vi "Laser Feedback-noglobalpower.vi"() -> ()   [LabVIEW 2014]
doc: "This VI first scan 0.1-5 V AOM voltage range 3 times, and use these data to generate a calibration curve. The calibration curve is fitted as a 3 th order polynomial curve, and then passed to the second part. \nSecond, the feedback loop is turned on and PID controller is used to stabilize the intensity.\n\nThis VI includes the following subVI:\n1. (SubVI)AOMvolt-Power Calibration.vi\n2. AOM PID feedback-simplePID(SubVI).vi"
uses:
  <vilib>/Analysis/polynomials.llb/Scalar Polynomial Evaluation (DBL).vi
  <vilib>/addons/control/pid/pid.llb/PID (DBL).vi
  <vilib>/Utility/file.llb/Write To Spreadsheet File (DBL).vi
  <vilib>/Analysis/NI_AALPro.lvlib
  <vilib>/addons/control/pid/NI_PID_pid.lvlib
panel:
  in  "Tab Control":enum32{"Calibration curve", "Power readout"}(tab)
  out "PW-AOM Graph":T1(graph)
  out "Waveform Chart":dbl(graph)
  out "Polynomial Coefficients":dbl[](array[numeric])
  out "AOM (V)":dbl format="%.2f"
  in  "Set Laser power":dbl
  out "Powermeter readout (mW)":dbl
  in  "Save Button":bool
  in  "PID gains 2":T2={"proportional gain (Kc)"=0.0091, "integral time (Ti, min)"=5e-06, "derivative time (Td, min)"=0.0014} {"derivative time (Td, min)" format="%#.6g"; "integral time (Ti, min)" format="%#.6g"; "proportional gain (Kc)" format="%#.6g"}
  in  "stop":bool
  in  "millisecond multiple":u32=5
  out "Start Calibrate":bool
  # "Kc=0.0151\nTi=2.1E-6\nTd=0.0093\n\nKc=0.0151\nTi=5E-6\nTd=0.0014"
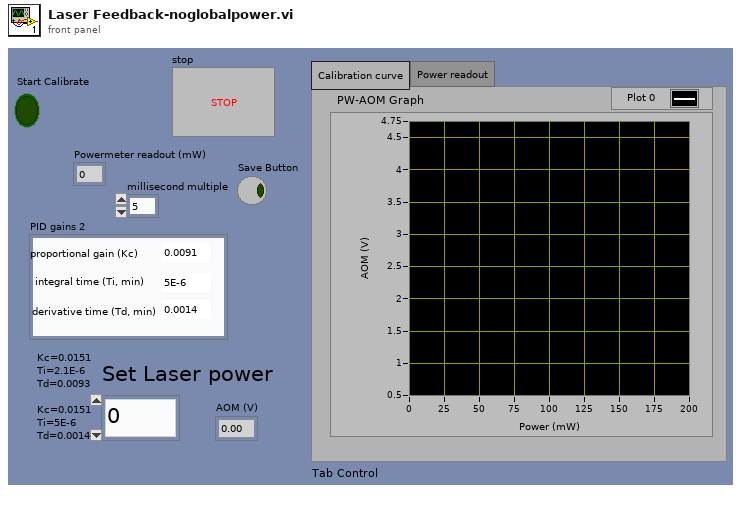
[diagram p1: front panel]
types:
  T1 = cluster{"Cal-PD (mV)":dbl[], "Cal-AOM (V)":dbl[]}[]
  T2 = cluster{"proportional gain (Kc)":dbl, "integral time (Ti, min)":dbl, "derivative time (Td, min)":dbl}
  T3 = cluster{"Cal-PD (mV)":dbl[], "Cal-AOM (V)":dbl[], "Best Polynomial Fit":dbl[], "Polynomial Coefficients":dbl[]}
  T4 = cluster{"Cal-PD (mV)":dbl[], "Best Polynomial Fit":dbl[]}
  T5 = cluster{"Cal-PD (mV)":dbl[], "Cal-AOM (V)":dbl[]}
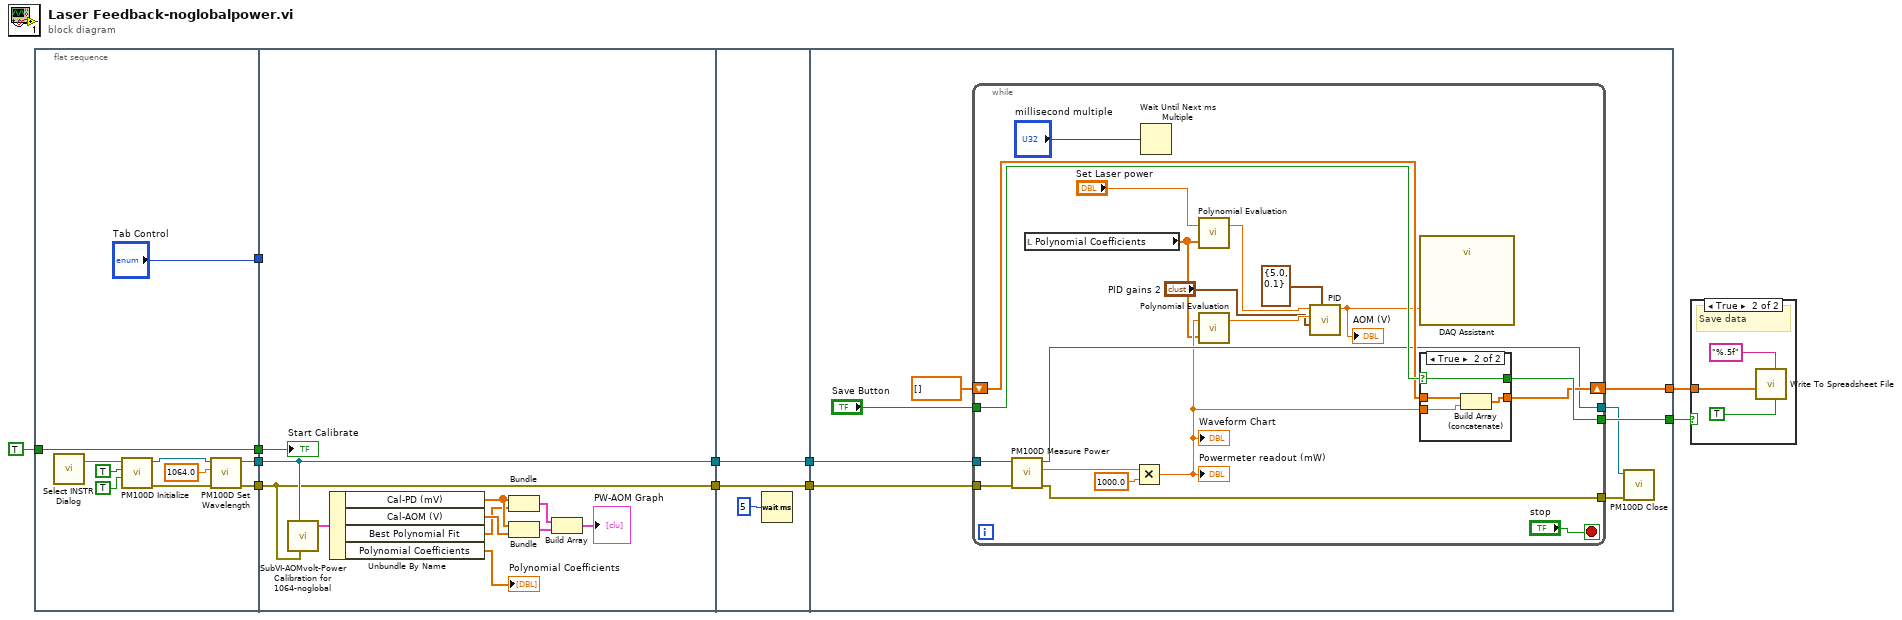
[diagram p0: block diagram]
diagram:
  n1 = flat-sequence {
    tunnel: TRUE -> [w21]
    tunnel: [w21] -> w10
    tunnel: [w14] -> w9
    tunnel: [w13] -> w8
    tunnel: ["Tab Control"] -> w1
    tunnel: w10 -> [w32]
    tunnel: w9 -> [w31]
    tunnel: w8 -> [w22]
    tunnel: [w31] -> w4
    tunnel: [w22] -> w2
    tunnel: w1 -> [_]
    tunnel: [w34] -> w5
    tunnel: w4 -> [w34]
    tunnel: [w33] -> w3
    tunnel: w2 -> [w33]
    tunnel: [w41] -> w7
    tunnel: [w40] -> w6
    tunnel: w5 -> [w39]
    tunnel: w3 -> [w38]
    frame #0 {
      n2 = call "Select INSTR Dialog.vi"() -> ("element"=w20:string)  [unwired: 1 in, 3 out]
      n3 = call <instrlib>:"PM100D Initialize.vi"("Reset Device (Reset Device)"=TRUE, "ID Query (Do Query)"=TRUE, "resource name"=w20) -> ("error out"=w17:errorcluster, "instrument handle out"=w15:refnum<visa-resource-name>)  [unwired: 7 in]
      n4 = call <instrlib>:"PM100D Set Wavelength.vi"("error in (no error)"=w17, "Wavelength (0.0)"=1064.0, "instrument handle"=w15) -> ("error out"=w13:errorcluster, "instrument handle out"=w14:refnum<visa-resource-name>)  [unwired: 7 in]
    }
    frame #1 {
      n5 = call "SubVI-AOMvolt-Power Calibration for 1064-noglobal.vi"("instrument handle"=w31, "error in (no error)"=w22) -> ("output cluster"=w30:T3)  [unwired: 5 in, 1 out]
      n6 = Unbundle By Name(w30) -> ("Cal-PD (mV)"=w27:dbl[], "Cal-AOM (V)"=w28:dbl[], "Best Polynomial Fit"=w26:dbl[], "Polynomial Coefficients"=→"Polynomial Coefficients":dbl[])
      n7 = Bundle("Cal-PD (mV)"=w27, "Best Polynomial Fit"=w26) -> (w25:T4)  [unwired: 1 in]
      n8 = Bundle("Cal-PD (mV)"=w27, "Cal-AOM (V)"=w28) -> (w24:T5)  [unwired: 1 in]
      n9 = Build Array(w25, w24) -> (→"PW-AOM Graph":T1)
      "Start Calibrate" <- w32
    }
    frame #2 {
      n10 = Wait (ms)(milliseconds to wait=u32 5) -> ()  [unwired: 1 out]
    }
    frame #3 {
      n11 = while {
        tunnel: "Save Button" -> [w58]
        tunnel: [w57] -> w41
        shift-right: [w56] -> w40
        shift-left: dbl[] [] -> [w55]
        tunnel: w39 -> [w51]
        tunnel: w38 -> [w50]
        tunnel: [w48] -> w37
        tunnel: [w47] -> w36
        stop <- "stop" stop-if-true
        n12 = call <instrlib>:"PM100D Measure Power.vi"("error in (no error)"=w50, "instrument handle"=w51) -> ("error out"=w47:errorcluster, "Power"=w52:dbl, "instrument handle out"=w48:refnum<visa-resource-name>)  [unwired: 7 in]
        n13 = local read "Polynomial Coefficients"() -> (w44:dbl[])
        n14 = Multiply(x=w52, y=1000.0) -> (x*y=w46:dbl)
        "Powermeter readout (mW)" <- w46
        "Waveform Chart" <- w46
        n15 = Wait Until Next ms Multiple(millisecond multiple="millisecond multiple") -> ()  [unwired: 1 out]
        n16 = call-poly <vilib>:"Polynomial Evaluation.vi"("P(x)"=w44, "a"="Set Laser power") -> ("P(a)"=w62:dbl)  [unwired: 1 out]
        n17 = call-poly <vilib>:"Polynomial Evaluation.vi"("P(x)"=w44, "a"=w46) -> ("P(a)"=w61:dbl)  [unwired: 1 out]
        n18 = call-poly <vilib>:"PID.vi"("output range"=cluster{"output high":dbl, "output low":dbl} {"output high"=5.0, "output low"=0.1}, "PID gains"="PID gains 2", "process variable"=w61, "setpoint"=w62) -> ("output"=w49:dbl)  [unwired: 6 in, 1 out]
        "AOM (V)" <- w49
        n19 = call "DAQ Assistant"("data"=w49) -> ()  [unwired: 17 in, 2 out]
        n20 = case shown="True" w58 {
          selector: w58 -> [w65 w69]
          tunnel: [w65 w69] -> w57
          tunnel: w46 -> [_ w67]
          tunnel: [w64 w66] -> w56
          tunnel: w55 -> [w64 w68]
          frame False {
          }
          frame True {
            n21 = Build Array (concatenate)(w68, w67) -> (w66:dbl[])
          }
        }
      }
      n22 = call <instrlib>:"PM100D Close.vi"("error in (no error)"=w36, "instrument handle"=w37) -> ()  [unwired: 9 in, 1 out]
    }
  }
  n23 = case shown="True" w7 {
    tunnel: w6 -> [_ w70]
    frame False {
    }
    frame True {
      # "Save data"
      n24 = call-poly <vilib>:"Write To Spreadsheet File.vi"("transpose? (no:F)"=TRUE, "format (%.3f)"="%.5f", "1D data"=w70) -> ()  [unwired: 5 in, 1 out]
    }
  }
